vi "Old_Ref2.vi"() -> ()   [LabVIEW 2020]
uses:
  <vilib>/Waveform/WDTOps.llb/WDT Waveform Duration DBL.vi
  <vilib>/Waveform/WDTOps.llb/WDT Get Waveform Subset DBL.vi
  <vilib>/measure/mamon.llb/Trigger Detection for 1 Channel.vi
  <vilib>/measure/mascope.llb/Transition Measurements 1 chan.vi
  <vilib>/measure/NI_MAPro.lvlib
  <vilib>/measure/mascope.llb/Pulse Measurements 1 chan.vi
panel:
  out "OG dt":dbl
  out "duration":dbl format="%e"
  out "actual start samples/time":dbl format="%e"
  out "ON Region":waveform(dbl)[](graph)
  out "NEW Tdon (ns)":dbl
  in  "reference  levels (CH1 initialize)":T1={"high ref level"=90.0, "mid ref level"=50.0, "low ref level"=10.0, "ref units"=1} {"ref units" items=["absolute", "percent"]; "high ref level" format="%0.2f"; "low ref level" format="%0.2f"; "mid ref level" format="%0.2f"}
  out "measurement info (CH2 1st Edge)":T2 {"ref levels"."ref units" items=["absolute", "relative"]; "ref levels"."high ref level" format="%.2p"; "ref levels"."low ref level" format="%.2p"; "ref levels"."mid ref level" format="%.2p"; "end time" format="%.6e"; "start time" format="%.6e"}
  in  "reference  levels (CH1 initialize)":T1={"high ref level"=90.0, "mid ref level"=50.0, "low ref level"=10.0, "ref units"=1} {"ref units" items=["absolute", "percent"]; "high ref level" format="%0.2f"; "low ref level" format="%0.2f"; "mid ref level" format="%0.2f"}
  out "measurement info (CH1 1st Edge)":T2 {"ref levels"."ref units" items=["absolute", "relative"]; "ref levels"."high ref level" format="%.2p"; "ref levels"."low ref level" format="%.2p"; "ref levels"."mid ref level" format="%.2p"; "end time" format="%.6e"; "start time" format="%.6e"}
  out "measurement info (CH1 2nd Edge)":T2 {"ref levels"."ref units" items=["absolute", "relative"]; "ref levels"."high ref level" format="%.2p"; "ref levels"."low ref level" format="%.2p"; "ref levels"."mid ref level" format="%.2p"; "end time" format="%.2p"; "start time" format="%.2p"}
  out "OLD Tdon (ns)":dbl format="%_6g"
  out "trigger location : 10% ICE":dbl format="%_7e"
  out "trigger location : 10% Vge":dbl format="%_7e"
  out "10% Ice":dbl
  out "10% Vge":dbl
  in  "ICE":dbl
  in  "VGE":dbl
  out "Waveform Graph":waveform(dbl)[](graph)
  out "error out":errorcluster
  in  "error in (no error)":errorcluster
  # "DUMMY 2 : Understanding  Waveform Graph"
  # "Tdon = From 10% Vge to 10% Ice"
  # "CursorFree deselect = off"
  # "Channel 2"
  # "Channel 1"
  # "Channel 2"
  # "Channel 1"
  # "Using absolute"
  # "56.3667"
  # "Using Percentage"
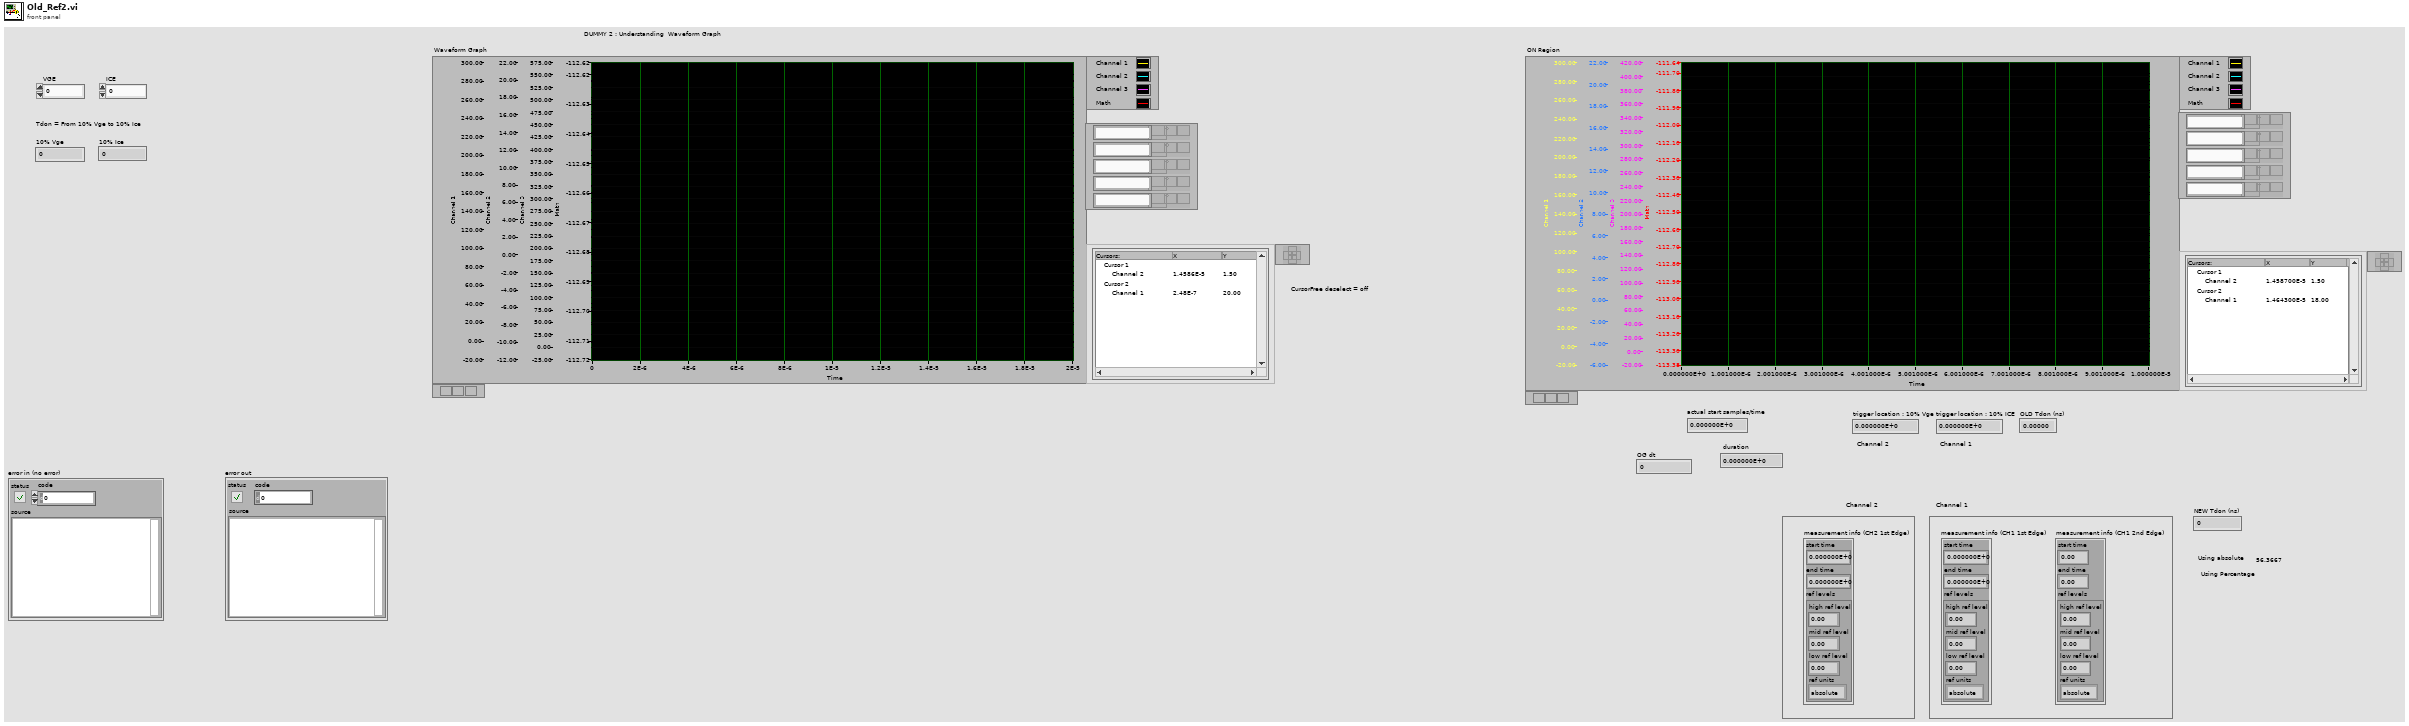
[diagram p1: front panel]
types:
  T1 = cluster{"high ref level":dbl, "mid ref level":dbl, "low ref level":dbl, "ref units":u16}
  T2 = cluster{"start time":dbl, "end time":dbl, "ref levels":cluster{"high ref level":dbl, "mid ref level":dbl, "low ref level":dbl, "ref units":u16}}
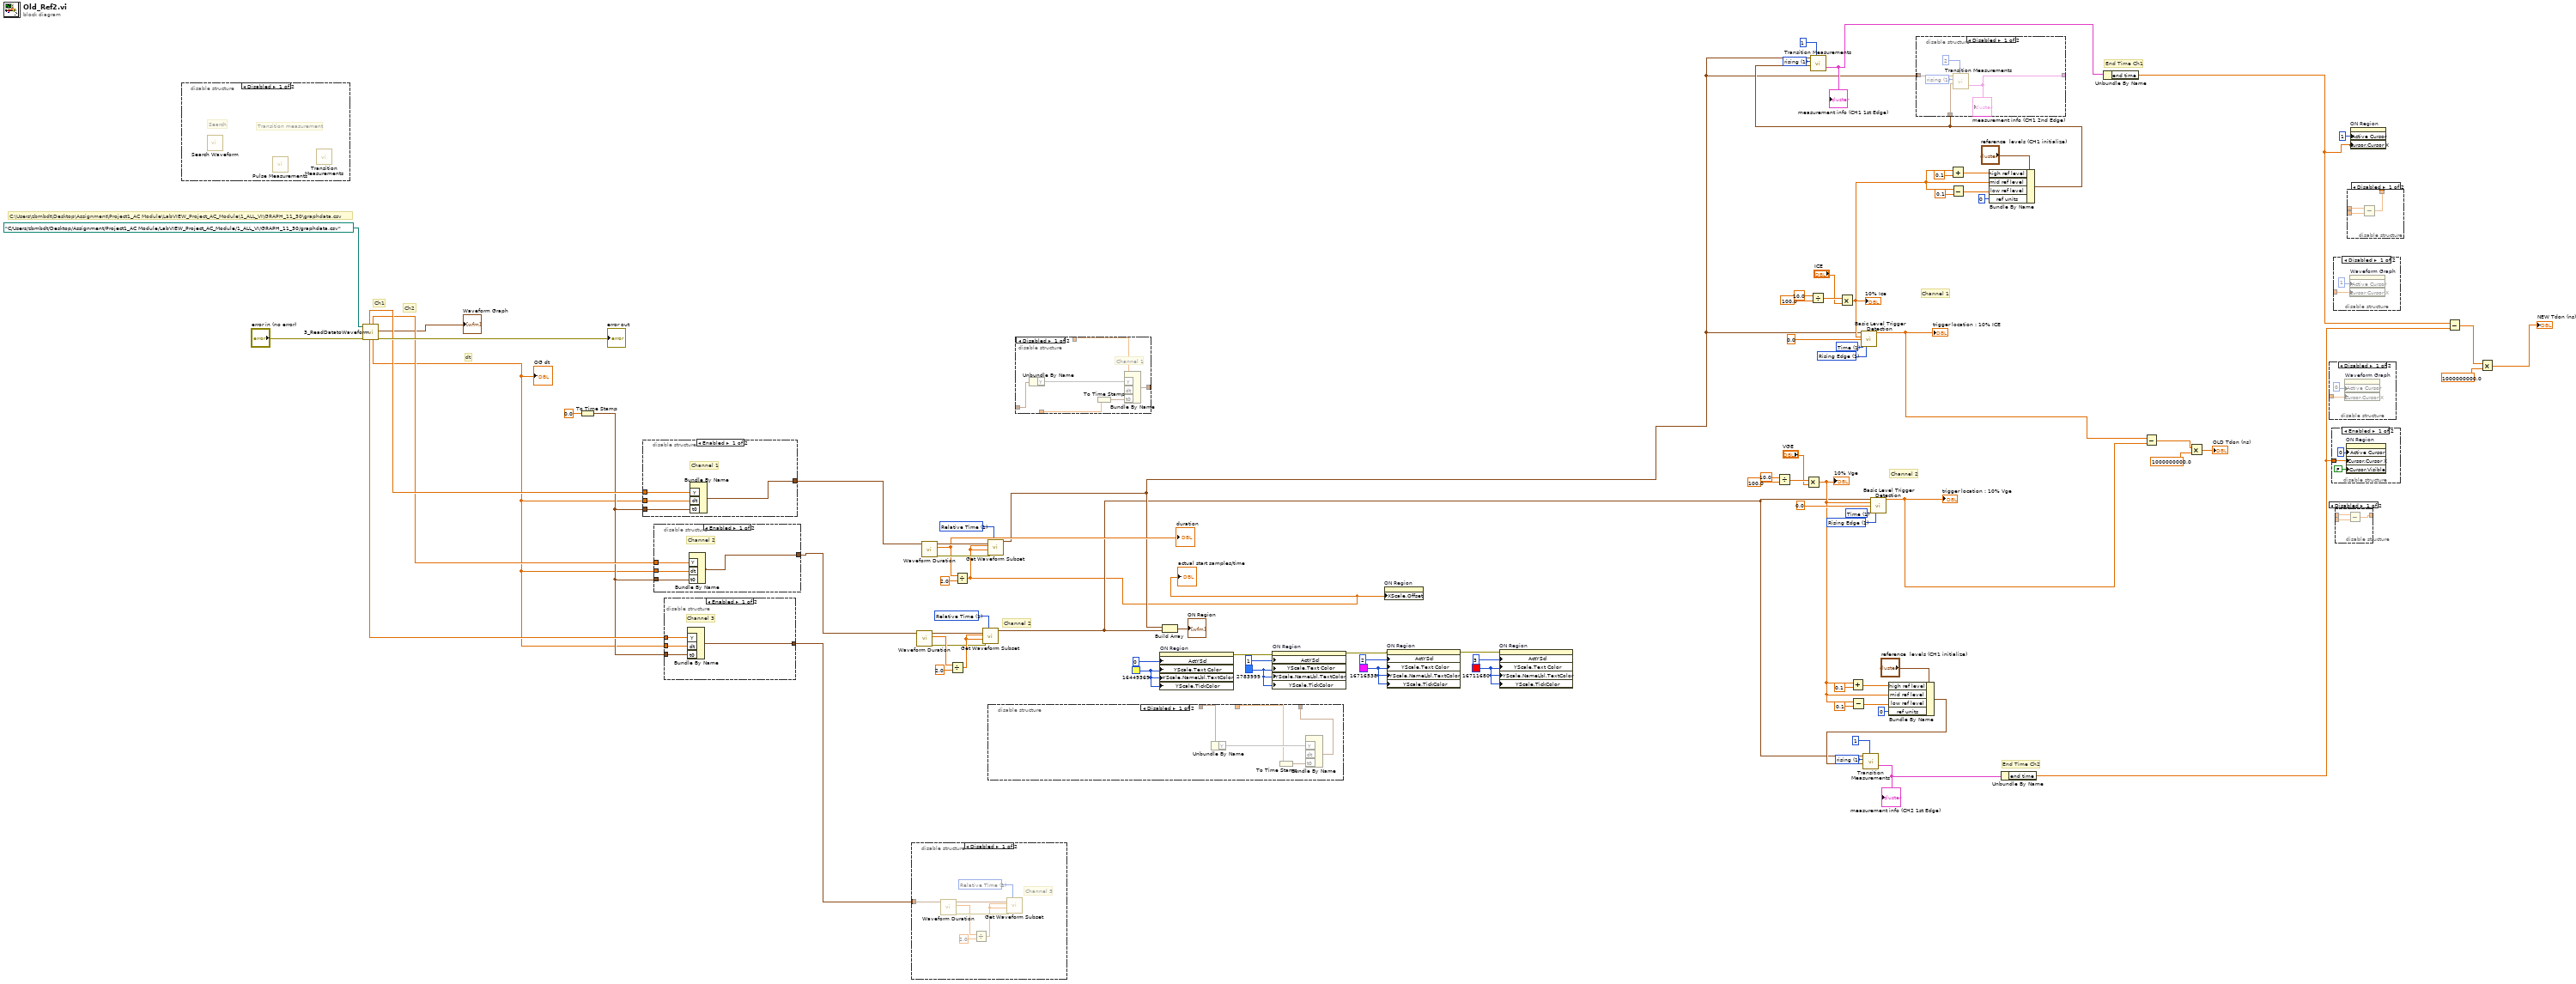
[diagram p0: block diagram]
diagram:
  w5 = u32 16711680 ("Y Scale.Marker Colors:Text Color")
  w6 = u32 16716538 ("Y Scale.Marker Colors:Text Color")
  w9 = u32 2783999 ("Y Scale.Marker Colors:Text Color")
  w10 = u32 16449369 ("Y Scale.Marker Colors:Text Color")
  w33 = u16 1 items=["Samples", "Relative Time"] ("start/duration format")
  w34 = u16 1 items=["Samples", "Relative Time"] ("start/duration format")
  w50 = u16 1 items=["falling", "rising"] ("polarity (rising)")
  w60 = u16 1 items=["falling", "rising"] ("polarity (rising)")
  w65 = u16 1 items=["Falling Edge", "Rising Edge"] ("trigger slope")
  w66 = u16 1 items=["Index", "Time"] ("location mode")
  w72 = u16 1 items=["Falling Edge", "Rising Edge"] ("trigger slope")
  w71 = u16 1 items=["Index", "Time"] ("location mode")
  # "Channel 2"
  # "End Time Ch2"
  # "End Time Ch1"
  # "Channel 2"
  # "Channel 1"
  # "Ch2"
  # "dt"
  # "Ch1"
  # "C:\\Users\\zbmbdt\\Desktop\\Assignment\\Project1_AC Module\\LabVIEW_Project_AC_Module\\1_ALL_VI\\GRAPH_11_30\\graphdata.csv"
  n1 = disable-structure shown="Disabled" {
    frame Disabled {
      # "Transition measurement"
      # "Search"
      n2 = call <vilib>:"Search Waveform.vi"() -> ()  [unwired: 6 in, 6 out]
      n3 = call-poly <vilib>:"Pulse Measurements.vi"() -> ()  [unwired: 7 in, 5 out]
      n4 = call-poly <vilib>:"Transition Measurements.vi"() -> ()  [unwired: 6 in, 6 out]
    }
    frame Enabled {
    }
  }
  n5 = call "3_ReadDatatoWaveform.vi"("error in (no error)"="error in (no error)", "file path (IN)"=path "C:/Users/zbmbdt/Desktop/Assignment/Project1_AC Module/LabVIEW_Project_AC_Module/1_ALL_VI/GRAPH_11_30/graphdata.csv") -> ("error out"=→"error out":errorcluster, "Waveform Graph"=→"Waveform Graph":waveform(dbl)[], "dt"=w20:dbl, "Ch 2 Data"=w74:dbl[], "Ch 3 Data"=w73:dbl[], "Ch 1 Data"=w75:dbl[])  [unwired: 3 in, 1 out]
  "OG dt" <- w20
  n6 = To Time Stamp(1:0.0 ("number")) -> (0:w69:timestamp)
  n7 = disable-structure shown="Enabled" {
    disable-tunnel: w69 -> [w90 _]
    disable-tunnel: w20 -> [w89 _]
    disable-tunnel: w75 -> [w88 _]
    disable-tunnel: [w87 _] -> w25
    frame Enabled {
      # "Channel 1"
      n8 = Bundle By Name("Y"=w88, "dt"=w89, "t0"=w90) -> (w87:waveform(dbl))  [unwired: 1 in]
    }
    frame Disabled {
    }
  }
  n9 = disable-structure shown="Enabled" {
    disable-tunnel: w69 -> [w94 _]
    disable-tunnel: w20 -> [w93 _]
    disable-tunnel: w74 -> [w92 _]
    disable-tunnel: [w91 _] -> w24
    frame Enabled {
      # "Channel 2"
      n10 = Bundle By Name("Y"=w92, "dt"=w93, "t0"=w94) -> (w91:waveform(dbl))  [unwired: 1 in]
    }
    frame Disabled {
    }
  }
  n11 = disable-structure shown="Enabled" {
    disable-tunnel: w69 -> [w98 _]
    disable-tunnel: w20 -> [w97 _]
    disable-tunnel: w73 -> [w96 _]
    disable-tunnel: [w95 _] -> w26
    frame Enabled {
      # "Channel 3"
      n12 = Bundle By Name("Y"=w96, "dt"=w97, "t0"=w98) -> (w95:waveform(dbl))  [unwired: 1 in]
    }
    frame Disabled {
    }
  }
  n13 = disable-structure shown="Disabled" {
    disable-tunnel: w26 -> [w99 _]
    frame Disabled {
      w100 = u16 1 items=["Samples", "Relative Time"] ("start/duration format")
      # "Channel 3"
      n14 = call-poly <vilib>:"Waveform Duration.vi"("waveform in"=w99) -> ("error out"=w105:errorcluster, "duration"=w102:dbl, "waveform out"=w104:waveform(dbl))  [unwired: 8 in]
      n15 = Divide(x=w102, y=2.0) -> (x/y=w101:dbl)
      n16 = call-poly <vilib>:"Get Waveform Subset.vi"("start/duration format"=w100, "error in (no error)"=w105, "duration"=w101, "start samples/time"=w101, "waveform in"=w104) -> ()  [unwired: 1 in, 4 out]
    }
    frame Enabled {
    }
  }
  n17 = call-poly <vilib>:"Waveform Duration.vi"("waveform in"=w24) -> ("error out"=w28:errorcluster, "duration"=w31:dbl, "waveform out"=w29:waveform(dbl))  [unwired: 8 in]
  n18 = call-poly <vilib>:"Waveform Duration.vi"("waveform in"=w25) -> ("error out"=w38:errorcluster, "duration"=w35:dbl, "waveform out"=w37:waveform(dbl))  [unwired: 8 in]
  "duration" <- w35
  n19 = Divide(x=w31, y=2.0) -> (x/y=w32:dbl)
  n20 = Divide(x=w35, y=2.0) -> (x/y=w18:dbl)
  "actual start samples/time" <- w18
  n21 = call-poly <vilib>:"Get Waveform Subset.vi"("start/duration format"=w33, "error in (no error)"=w28, "duration"=w32, "start samples/time"=w32, "waveform in"=w29) -> ("waveform out"=w19:waveform(dbl))  [unwired: 1 in, 3 out]
  n22 = call-poly <vilib>:"Get Waveform Subset.vi"("start/duration format"=w34, "error in (no error)"=w38, "duration"=w18, "start samples/time"=w18, "waveform in"=w37) -> ("waveform out"=w21:waveform(dbl))  [unwired: 1 in, 3 out]
  n23 = disable-structure shown="Disabled" {
    disable-tunnel: _ -> [w109 _]
    disable-tunnel: [w108 _] -> _
    disable-tunnel: _ -> [w107 _]
    frame Disabled {
      n24 = Unbundle By Name(w109) -> ("Y"=w111)
      n25 = To Time Stamp(1:w107) -> (0:w110:timestamp)
      n26 = Bundle By Name("Y"=w111, "t0"=w110) -> (w108:waveform(dbl), "dt"=w106:dbl)  [unwired: 1 in]
    }
    frame Enabled {
    }
  }
  n27 = disable-structure shown="Disabled" {
    disable-tunnel: _ -> [w117 _]
    disable-tunnel: [w114 _] -> _
    disable-tunnel: _ -> [w113 _]
    disable-tunnel: _ -> [w112 _]
    frame Disabled {
      # "Channel 1"
      n28 = Unbundle By Name(w117) -> ("Y"=w116)
      n29 = To Time Stamp(1:w112) -> (0:w115:timestamp)
      n30 = Bundle By Name("Y"=w116, "dt"=w113, "t0"=w115) -> (w114:waveform(dbl))  [unwired: 1 in]
    }
    frame Enabled {
    }
  }
  n31 = property on="ON Region" class="WFGraph (strict)"("ActYScl"=0 ("Active Y Scale"), "YScale.Text Color"=w10, "YScale.NameLbl.TextColor"=w10, "YScale.TickColor"=w10) -> (error out=w3:errorcluster)  [unwired: 2 in, 1 out]
  n32 = Build Array(w21, w19) -> (→"ON Region":waveform(dbl)[])
  n33 = property on="ON Region" class="WFGraph (strict)"(error in=w3, "ActYScl"=1 ("Active Y Scale"), "YScale.Text Color"=w9, "YScale.NameLbl.TextColor"=w9, "YScale.TickColor"=w9) -> (error out=w2:errorcluster)  [unwired: 1 in, 1 out]
  n34 = property on="ON Region" class="WFGraph (strict)"("XScale.Offset"=w18) -> ()  [unwired: 2 in, 2 out]
  n35 = property on="ON Region" class="WFGraph (strict)"(error in=w2, "ActYScl"=2 ("Active Y Scale"), "YScale.Text Color"=w6, "YScale.NameLbl.TextColor"=w6, "YScale.TickColor"=w6) -> (error out=w1:errorcluster)  [unwired: 1 in, 1 out]
  n36 = property on="ON Region" class="WFGraph (strict)"(error in=w1, "ActYScl"=3 ("Active Y Scale"), "YScale.Text Color"=w5, "YScale.NameLbl.TextColor"=w5, "YScale.TickColor"=w5) -> ()  [unwired: 1 in, 2 out]
  n37 = Divide(x=10.0, y=100.0) -> (x/y=w83:dbl)
  n38 = Multiply(x=w83, y="VGE") -> (x*y=w41:dbl)
  "10% Vge" <- w41
  n39 = Divide(x=10.0, y=100.0) -> (x/y=w81:dbl)
  n40 = Multiply(x=w81, y="ICE") -> (x*y=w56:dbl)
  "10% Ice" <- w56
  n41 = Add(x=w41, y=0.1) -> (x+y=w46:dbl)
  n42 = Subtract(x=w41, y=0.1) -> (x-y=w45:dbl)
  n43 = call-poly <vilib>:"Basic Level Trigger Detection.vi"("signal in"=w21, "level"=w56, "hysteresis"=0.0, "location mode"=w66, "trigger slope"=w65) -> ("trigger location"=w64:dbl)  [unwired: 8 in, 2 out]
  "trigger location : 10% ICE" <- w64
  n44 = call-poly <vilib>:"Basic Level Trigger Detection.vi"("signal in"=w19, "level"=w41, "hysteresis"=0.0, "location mode"=w71, "trigger slope"=w72) -> ("trigger location"=w12:dbl)  [unwired: 8 in, 2 out]
  "trigger location : 10% Vge" <- w12
  n45 = Bundle By Name(cluster="reference  levels (CH1 initialize)", "high ref level"=w46, "mid ref level"=w41, "low ref level"=w45, "ref units"=u16 0) -> (w42:T1)
  n46 = call-poly <vilib>:"Transition Measurements.vi"("edge number (1)"=1, "reference levels"=w42, "polarity (rising)"=w50, "signal in"=w19) -> ("measurement info"=w40:T2)  [unwired: 2 in, 5 out]
  "measurement info (CH2 1st Edge)" <- w40
  n47 = Add(x=w56, y=0.1) -> (x+y=w55:dbl)
  n48 = Subtract(x=w56, y=0.1) -> (x-y=w54:dbl)
  n49 = Bundle By Name(cluster="reference  levels (CH1 initialize)", "high ref level"=w55, "mid ref level"=w56, "low ref level"=w54, "ref units"=u16 0) -> (w49:T1)
  n50 = call-poly <vilib>:"Transition Measurements.vi"("edge number (1)"=1, "reference levels"=w49, "polarity (rising)"=w60, "signal in"=w21) -> ("measurement info"=w22:T2)  [unwired: 2 in, 5 out]
  "measurement info (CH1 1st Edge)" <- w22
  n51 = disable-structure shown="Disabled" {
    disable-tunnel: w49 -> [w120 _]
    disable-tunnel: [w119 _] -> _
    disable-tunnel: w21 -> [w118 _]
    frame Disabled {
      w121 = u16 1 items=["falling", "rising"] ("polarity (rising)")
      n52 = call-poly <vilib>:"Transition Measurements.vi"("edge number (1)"=2, "reference levels"=w120, "polarity (rising)"=w121, "signal in"=w118) -> ("measurement info"=w119:T2)  [unwired: 2 in, 5 out]
      "measurement info (CH1 2nd Edge)" <- w119
    }
    frame Enabled {
    }
  }
  n53 = Unbundle By Name(w40) -> ("end time"=w17:dbl)
  n54 = Unbundle By Name(w22) -> ("end time"=w16:dbl)
  n55 = Subtract(x=w64, y=w12) -> (x-y=w63:dbl)
  n56 = Multiply(x=w63, y=1000000000.0) -> (x*y=→"OLD Tdon (ns)":dbl)
  n57 = disable-structure shown="Disabled" {
    disable-tunnel: _ -> [w123 _]
    frame Disabled {
      n58 = property on="Waveform Graph" class="WFGraph (strict)"("Active Cursor"=u32 0, "Cursor.Cursor X"=w123) -> ()  [unwired: 2 in, 2 out]
    }
    frame Enabled {
    }
  }
  n59 = disable-structure shown="Enabled" {
    disable-tunnel: w17 -> [w126 _]
    frame Enabled {
      n60 = property on="ON Region" class="WFGraph (strict)"("Active Cursor"=u32 0, "Cursor.Cursor X"=w126, "Cursor.Visible"=FALSE) -> ()  [unwired: 2 in, 2 out]
    }
    frame Disabled {
    }
  }
  n61 = disable-structure shown="Disabled" {
    disable-tunnel: _ -> [w128 _]
    frame Disabled {
      n62 = property on="Waveform Graph" class="WFGraph (strict)"("Active Cursor"=u32 1, "Cursor.Cursor X"=w128) -> ()  [unwired: 2 in, 2 out]
    }
    frame Enabled {
    }
  }
  n63 = disable-structure shown="Disabled" {
    disable-tunnel: _ -> [w132 _]
    disable-tunnel: [w131 _] -> _
    disable-tunnel: _ -> [w130 _]
    frame Disabled {
      n64 = Subtract(x=w132, y=w130) -> (x-y=w131:dbl)
    }
    frame Enabled {
    }
  }
  n65 = disable-structure shown="Disabled" {
    disable-tunnel: [w135 _] -> _
    disable-tunnel: _ -> [w134 _]
    disable-tunnel: _ -> [w133 _]
    frame Disabled {
      n66 = Subtract(x=w134, y=w133) -> (x-y=w135:dbl)
    }
    frame Enabled {
    }
  }
  n67 = property on="ON Region" class="WFGraph (strict)"("Active Cursor"=u32 1, "Cursor.Cursor X"=w16) -> ()  [unwired: 2 in, 2 out]
  n68 = Subtract(x=w16, y=w17) -> (x-y=w14:dbl)
  n69 = Multiply(x=w14, y=1000000000.0) -> (x*y=→"NEW Tdon (ns)":dbl)
